vi "Get-abort.vi"(8 "error in (no error)":errorcluster, 11 "Object ref in":T1) -> (0 "error out":errorcluster, 2 "Abort":bool, 3 "Object ref out":T1)   [LabVIEW 2013, in "SLMControl.lvlib" / "SC-Main.lvclass"]
uses:
  SC-Main.lvclass
  Object-reference.ctl
  SC-Main.lvclass/SC-Main.ctl
  Read Abort.vi
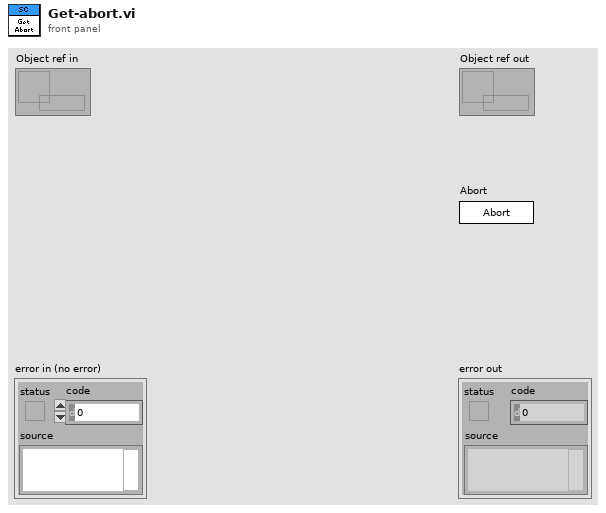
[diagram p1: front panel]
types:
  T1 = typedef "SLMControl.lvlib/SC-Main.lvclass/Object-reference.ctl" = refnum<data-value>
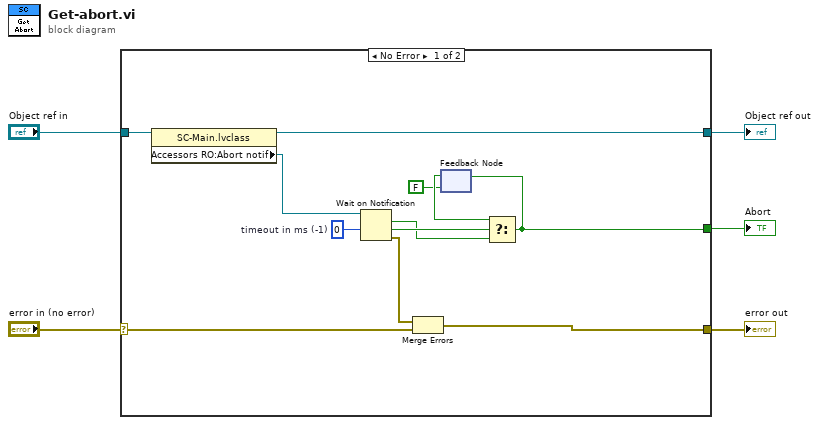
[diagram p0: block diagram]
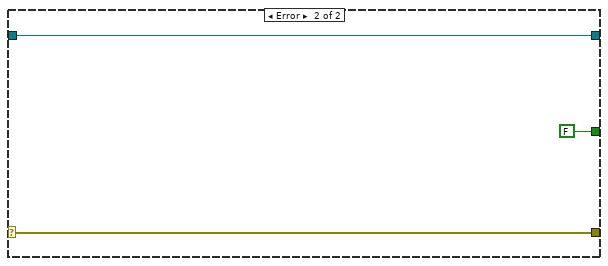
[diagram p2: hidden frame]
diagram:
  n1 = case shown="No Error" "error in (no error)" {
    selector: "error in (no error)" -> [w6 w20]
    tunnel: [w7 w20] -> w4
    tunnel: [w16 w19] -> w2
    tunnel: "Object ref in" -> [w17 w19]
    tunnel: [w8 FALSE] -> w1
    frame No Error {
      w13 = 0  # timeout in ms (-1)
      n2 = property class="SC-Main.lvclass"(reference=w17) -> (reference out=w16:T1, "Accessors RO:Abort notif"=w15:refnum<notifier>)  [unwired: 1 in, 1 out]
      n3 = Wait on Notification(notifier=w15, timeout in ms (-1)=w13) -> (notification=w11:bool, timed out?=w12:bool, error out=w14:errorcluster)  [unwired: 2 in, 1 out]
      n4 = Merge Errors(w14, w6) -> (w7:errorcluster)
      n5 = feedback #1(FALSE) -> (w10:bool)
      n6 = Select(t=w10, s=w12, f=w11) -> (s? t:f=w8:bool)
      n7 = feedback-in #1(w8) -> ()
    }
    frame Error {
    }
  }
  "error out" <- w4
  "Object ref out" <- w2
  "Abort" <- w1
